vi "subVI.vi"(11 "String":string) -> (3 "numeri":dbl[](array[numeric]))   [LabVIEW 2013]
panel:
  out "error out":errorcluster
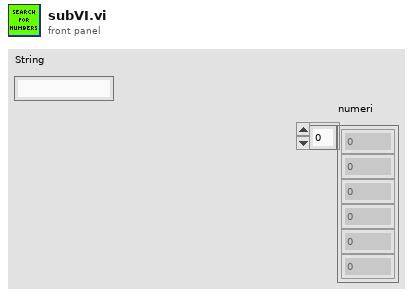
[diagram p1: front panel]
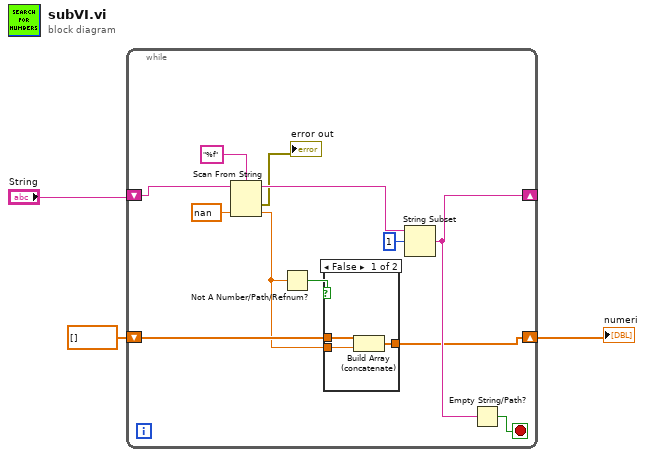
[diagram p0: block diagram]
diagram:
  n1 = while {
    shift-right: [w8] -> _
    shift-left: "String" -> [w10]
    shift-right: [w6] -> w2
    shift-left: dbl[] [] -> [w7]
    stop <- w9 stop-if-true
    n2 = Scan From String(format string="%f", input string=w10, default 1=nan ("default value 1")) -> (remaining string=w14:string, error out=→"error out":errorcluster, output 1=w4:dbl)  [unwired: 2 in, 1 out]
    n3 = Not A Number/Path/Refnum?(number/path/refnum=w4) -> (NaN/Path/Refnum?=w5:bool)
    n4 = case shown="False" w5 {
      tunnel: w4 -> [w18 _]
      tunnel: w7 -> [w17 w19]
      tunnel: [w16 w19] -> w6
      frame False {
        n5 = Build Array (concatenate)(w17, w18) -> (w16:dbl[])
      }
      frame True {
      }
    }
    n6 = String Subset(string=w14, offset (0)=1) -> (substring=w8:string)  [unwired: 1 in]
    n7 = Empty String/Path?(string/path=w8) -> (empty?=w9:bool)
  }
  "numeri" <- w2
